vi "Test Binary Serialisation With Classes.vi"() -> ()   [LabVIEW 2021]
uses:
  Source/Abs_Types/Boolean/Abs_Boolean.lvclass
panel:
  out "Binary 5":string
  out "Boolean 2":bool
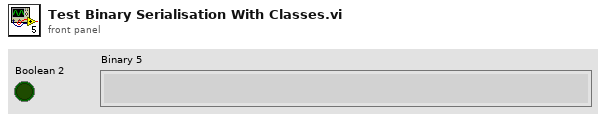
[diagram p1: front panel]
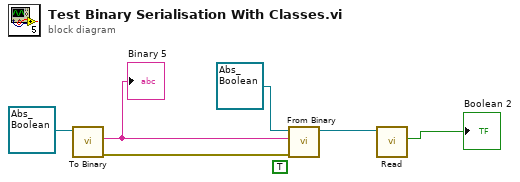
[diagram p0: block diagram]
diagram:
  (unwired) TRUE ("Class Name is Included")
  n1 = call-dynamic "To Binary.vi"("Boolean in"=refnum<class "Abs_Boolean.lvclass"> refnum) -> ("error out"=w6:errorcluster, "Binary"=w5:string)  [unwired: 8 in, 1 out]
  "Binary 5" <- w5
  n2 = call-dynamic "From Binary.vi"("error in (no error)"=w6, "Binary"=w5, "Boolean in"=refnum<class "Abs_Boolean.lvclass"> refnum) -> ("Boolean out"=w4:refnum<class "Abs_Boolean.lvclass">)  [unwired: 6 in, 2 out]
  n3 = call-dynamic "Read.vi"("Boolean in"=w4) -> ("Boolean"=→"Boolean 2":bool)  [unwired: 8 in, 2 out]
